vi "hmi-programming.vi"() -> ()   [LabVIEW 2017]
doc: "Demonstrates how to write and receive CAN frames via the Network Interface on the same port. \n\nTo write and receive frames via the Network Interface:\n- select the CAN Network Interface (i.e. CAN0, CAN1, etc.)\n- select the Baud Rate\n- run the VI\n- press the write button to write frames to the can bus\n\nEnable RTR Button to send a Remote Transmission Request or to simply send an empty Frame to request an Answer Frame from a connected device.\n\nEnable Extended Button to write extended Identifier Format. This is done by setting the 30th bit to enable extended format with the driver."
uses:
  <vilib>/nican/nican.llb/ncNetAttr.ctl
panel:
  in  "Tab Control":enum32{"Program", "Settings"}(tab)
  out "ID":u16 format="%04x"
  in  "Device":enum16{"Device 1", "Device 2"}(ring)
  out "Heartbeat":u16 format="%04x"
  in  "binFile":path
  in  "shutdown":bool
  in  "Initialize DFU":bool
  in  "Program":bool
  out "DFU Ready":bool
  out "Valid Path":bool
  out "Normal":bool
  in  "interface":string(combo)="CAN0" caption="Interface"
  # "PRESS AND HOLD"
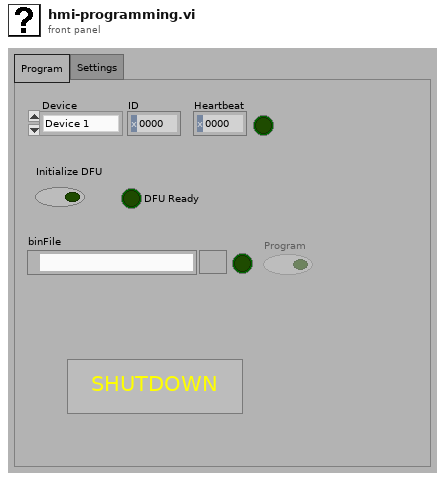
[diagram p1: front panel]
types:
  T1 = cluster{"Heartbeat":u16, "DFU":bool, "ValidPath":bool, "Path":path, "Normal":bool}
  T2 = typedef "ncNetAttr.ctl" = cluster{"Start On Open":enum32{"FALSE", "TRUE"}, "Baud Rate":u32, "Read Queue Length":u32, "Write Queue Length":u32, "Standard Comparator":u32, "Standard Mask":u32, "Extended Comparator":u32, "Extended Mask":u32}
  T3 = typedef "xobjhandle.ctl" = u32
  T4 = enum8{"Enabled", "Disabled", "Disabled and Grayed Out"}
  T5 = typedef "CanFrameTimed.ctl" = cluster{"Timestamp":dbl, "ArbitrationId":u32, "IsRemote":u8, "DataLength":u8, "Data":u8[]}
  T6 = cluster{dbl, u32, "IsRemote":u8, "DataLength":u8, u8[]}
  T7 = cluster{dbl, u32, "IsRemote":u8, "DataLength":u8, u8[]}[]
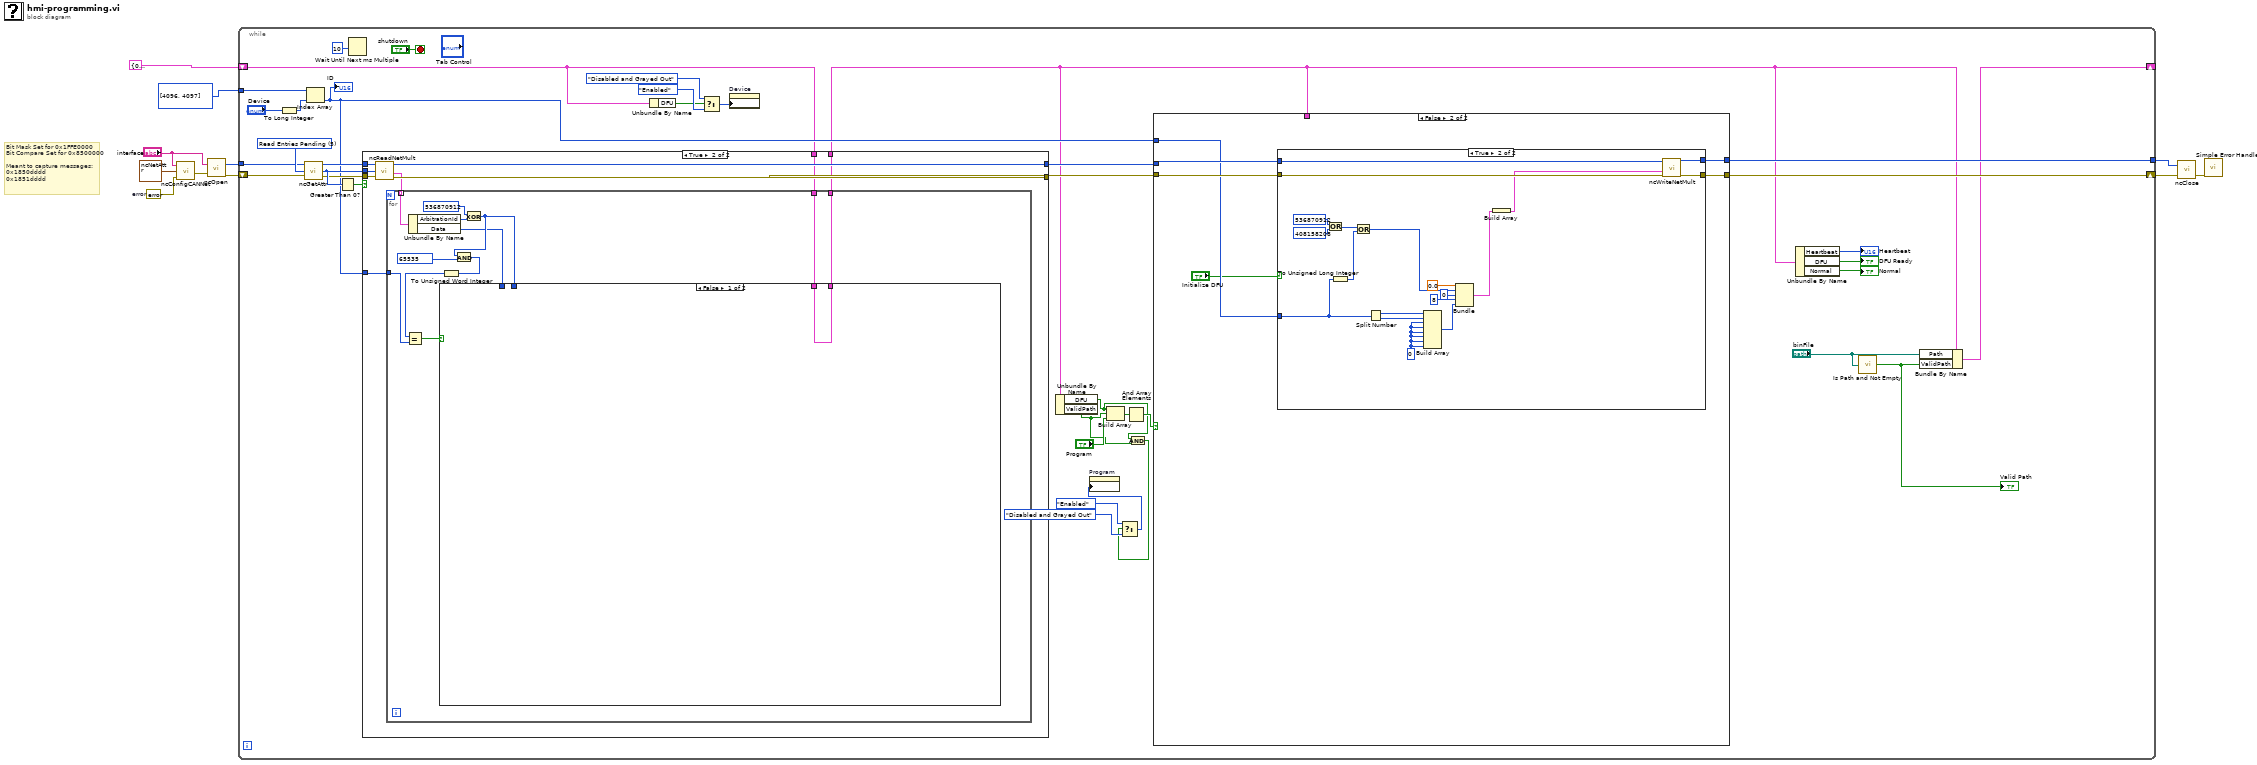
[diagram p0: block diagram]
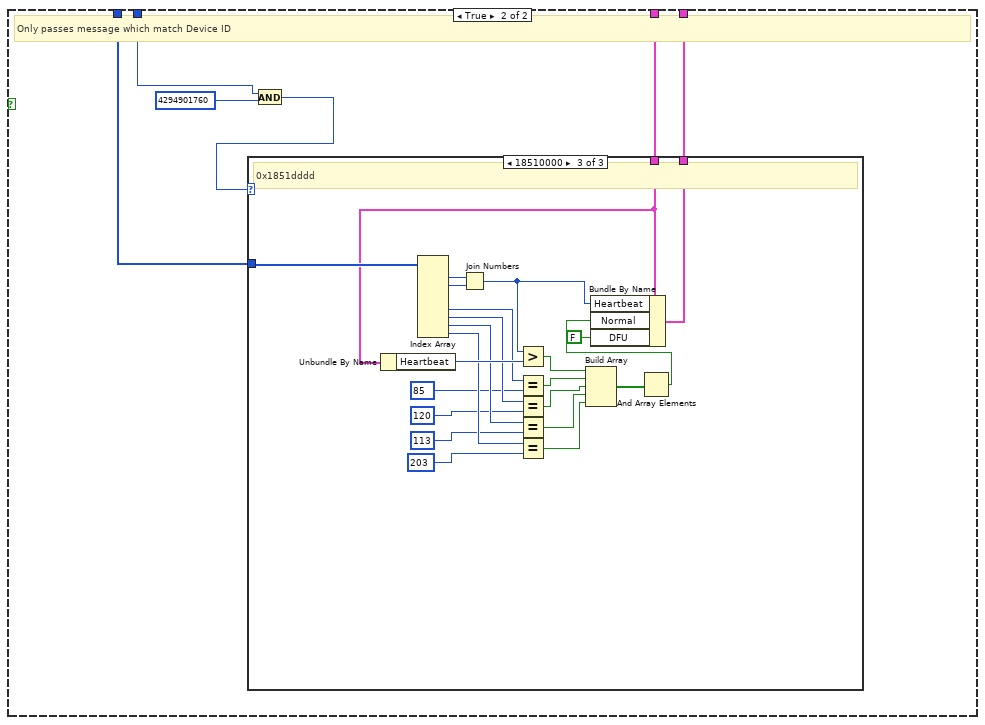
[diagram p3: hidden frame]
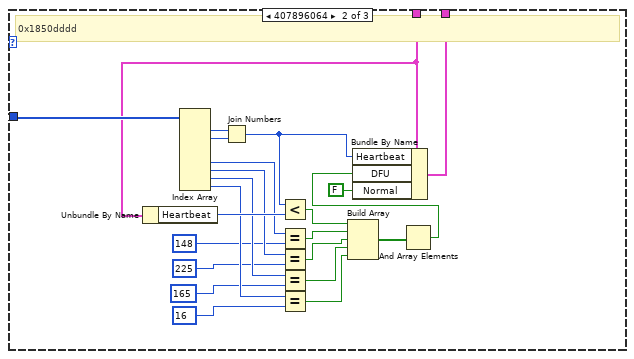
[diagram p5: hidden frame]
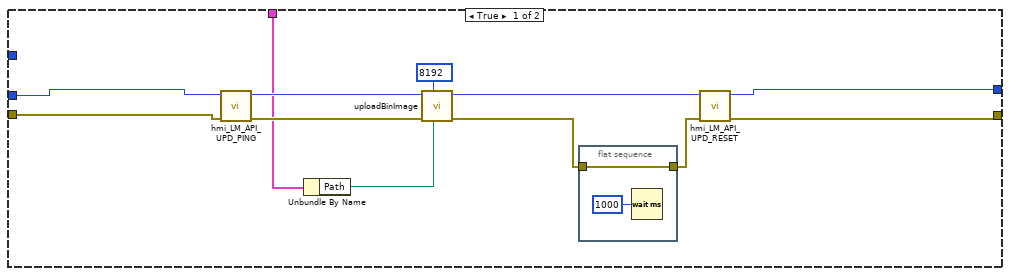
[diagram p6: hidden frame]
diagram:
  w7 = errorcluster {"status"=FALSE, "code"=0, "source"=""}  # error
  # "Bit Mask Set for 0x1FFE0000\nBit Compare Set for 0x8500000\n\nMeant to capture messages:\n0x1850dddd\n0x1851dddd"
  n1 = call <vilib>:"ncConfigCANNet.vi"("Error in"=w7, "CAN Network Interface Config"=T2 {"Start On Open"=enum."TRUE", "Baud Rate"=1000000, "Read Queue Length"=150, "Write Queue Length"=150, "Standard Comparator"=0, "Standard Mask"=0, "Extended Comparator"=407896064, "Extended Mask"=536739840}, "ObjName"="interface") -> ("Error out"=w8:errorcluster)  [unwired: 2 in]
  n2 = call <vilib>:"ncOpen.vi"("Error in"=w8, "ObjName"="interface") -> ("Error out"=w11:errorcluster, "ObjHandle out"=w9:T3)
  n3 = while {
    tunnel: w9 -> [w38]
    tunnel: [w48] -> w4
    shift-right: [w49] -> w3
    shift-left: w11 -> [w37]
    tunnel: u16[] [4096, 4097] -> [w36]
    shift-right: [w26] -> _
    shift-left: T1 {"Heartbeat"=0, "DFU"=FALSE, "ValidPath"=FALSE, "Path"=path "", "Normal"=FALSE} -> [w19]
    stop <- "shutdown" stop-if-true
    w41 = u32 5 items=["(reserved)", "Protocol Version", "Software Version", "Object State", "(reserved)", "Read Entries Pending", "Write Entries Pending", "ReadMult Size for Notification", "Listen Only?", "Self Reception?", "Transmit Error Counter", "Receive Error Counter", "Single Shot Transmit?", "Series 2 Filter Mode", "Series 2 Mask", "Series 2 Comparator", "Serial Number", "Form Factor", "Series", "Transceiver Type", "Interface Number", "Series 2 Error/Arb Capture", "Transceiver Mode", "Transceiver External Outputs", "Transceiver External Inputs", "Start Trigger Behavior", "Log Comm Warnings", "User RTSI Frame", "Transmit Mode", "Log Start Trigger?", "Timestamp Format", "Master Timebase Rate", "Virtual Bus Timing"] ("AttrId")
    n4 = To Long Integer(number="Device") -> (32bit integer=w34:i32)
    n5 = call <vilib>:"ncGetAttr.vi"("Error in"=w37, "AttrId"=w41, "ObjHandle in"=w38) -> ("Error out"=w42:errorcluster, "AttrValue"=w45:u32, "ObjHandle out"=w43:T3)
    n6 = Index Array(array=w36, index=w34) -> (element=w33:u16)
    "ID" <- w33
    n7 = Greater Than 0?(x=w45) -> (x > 0?=w44:bool)
    n8 = Wait Until Next ms Multiple(millisecond multiple=u32 10) -> ()  [unwired: 1 out]
    n9 = case shown="True" w44 {
      tunnel: [w51 w61] -> w39
      tunnel: [w52 w60] -> w40
      tunnel: w45 -> [_ w59]
      tunnel: w42 -> [w51 w58]
      tunnel: w43 -> [w52 w57]
      tunnel: w33 -> [_ w55]
      tunnel: w19 -> [w50 w54]
      tunnel: [w50 w53] -> w27
      frame False {
      }
      frame True {
        n10 = call <vilib>:"ncReadNetMult.vi"("ObjHandle in"=w57, "Requested Number of Frames"=w59, "Error in"=w58) -> ("ObjHandle out"=w60:T3, "Data"=w56:T5[], "Error out"=w61:errorcluster)  [unwired: 1 out]
        n11 = for {
          tunnel: w56 -> [w73] mode=indexing
          tunnel: w55 -> [w70]
          tunnel: w54 -> [w64]
          tunnel: [w63] -> w53
          n12 = Unbundle By Name(w73) -> ("ArbitrationId"=w71:u32, "Data"=w66:u8[])
          n13 = Exclusive Or(1:w71, 2:u32 536870912 ("y")) -> (0:w67:u32)
          n14 = And(x=w67, y=u32 65535) -> (x .and. y?=w69:u32)
          n15 = To Unsigned Word Integer(number=w69) -> (unsigned 16bit integer=w65:u16)
          n16 = Equal?(x=w65, y=w70) -> (x = y?=w68:bool)
          n17 = case shown="False" w68 {
            tunnel: w67 -> [_ w75]
            tunnel: w66 -> [_ w80]
            tunnel: w64 -> [w74 w78]
            tunnel: [w74 w77] -> w63
            frame False {
            }
            frame True {
              # "Only passes message which match Device ID"
              n18 = And(x=w75, y=u32 4294901760) -> (x .and. y?=w79:u32)
              n19 = case shown="18510000" w79 {
                tunnel: w80 -> [_ w102 w125]
                tunnel: w78 -> [w81 w100 w123]
                tunnel: [w81 w101 w124] -> w77
                frame Default {
                }
                frame 407896064 {
                  # "0x1850dddd"
                  n20 = Unbundle By Name(w100) -> ("Heartbeat"=w99:u16)
                  n21 = Index Array(array=w102) -> (element #1=w103:u8, element #2=w104:u8, element #5=w92:u8, element #6=w91:u8, element #7=w90:u8, element #8=w89:u8)  [unwired: 8 in, 2 out]
                  n22 = Join Numbers(hi=w103, lo=w104) -> ((hi.lo)=w98:u16)
                  n23 = Less?(x=w98, y=w99) -> (x < y?=w97:bool)
                  n24 = Equal?(x=w92, y=u8 148) -> (x = y?=w96:bool)
                  n25 = Equal?(x=w91, y=u8 225) -> (x = y?=w95:bool)
                  n26 = Equal?(x=w90, y=u8 165) -> (x = y?=w94:bool)
                  n27 = Equal?(x=w89, y=u8 16) -> (x = y?=w93:bool)
                  n28 = Build Array(w97, w96, w95, w94, w93) -> (w84:bool[])
                  n29 = And Array Elements(Boolean array=w84) -> (logical AND=w83:bool)
                  n30 = Bundle By Name(cluster=w100, "Heartbeat"=w98, "DFU"=w83, "Normal"=FALSE) -> (w101:T1)
                }
                frame 407961600 {
                  # "0x1851dddd"
                  n31 = Unbundle By Name(w123) -> ("Heartbeat"=w122:u16)
                  n32 = Index Array(array=w125) -> (element #1=w126:u8, element #2=w127:u8, element #5=w115:u8, element #6=w114:u8, element #7=w113:u8, element #8=w112:u8)  [unwired: 8 in, 2 out]
                  n33 = Join Numbers(hi=w126, lo=w127) -> ((hi.lo)=w121:u16)
                  n34 = Greater?(x=w121, y=w122) -> (0:w120:bool)
                  n35 = Equal?(x=w115, y=u8 85) -> (x = y?=w119:bool)
                  n36 = Equal?(x=w114, y=u8 120) -> (x = y?=w118:bool)
                  n37 = Equal?(x=w113, y=u8 113) -> (x = y?=w117:bool)
                  n38 = Equal?(x=w112, y=u8 203) -> (x = y?=w116:bool)
                  n39 = Build Array(w120, w119, w118, w117, w116) -> (w107:bool[])
                  n40 = And Array Elements(Boolean array=w107) -> (logical AND=w106:bool)
                  n41 = Bundle By Name(cluster=w123, "Heartbeat"=w121, "Normal"=w106, "DFU"=FALSE) -> (w124:T1)
                }
              }
            }
          }
        }
      }
    }
    n42 = Unbundle By Name(w19) -> ("DFU"=w18:bool)
    n43 = Select(t=T4."Disabled and Grayed Out" ("Disabled"), s=w18, f=T4."Enabled" ("Disabled")) -> (s? t:f=w20:T4)
    n44 = property on="Device" class="Enum (strict)"("DisabledEnum"=w20) -> ()  [unwired: 2 in, 2 out]
    n45 = Unbundle By Name(w27) -> ("DFU"=w14:bool, "ValidPath"=w13:bool)
    n46 = Build Array(w14, w13, "Program") -> (w29:bool[])
    n47 = And Array Elements(Boolean array=w29) -> (logical AND=w28:bool)
    n48 = And(x=w14, y=w13) -> (x .and. y?=w12:bool)
    n49 = Select(t=T4."Enabled" ("Disabled"), s=w12, f=T4."Disabled and Grayed Out" ("Disabled")) -> (s? t:f=w15:T4)
    n50 = property on="Program" class="Bool"("DisabledEnum"=w15) -> ()  [unwired: 2 in, 2 out]
    n51 = case shown="False" w28 {
      tunnel: [w130 w147] -> w49
      tunnel: [w131 w146] -> w48
      tunnel: w40 -> [w133 w145]
      tunnel: w39 -> [w132 w144]
      tunnel: w33 -> [_ w143]
      tunnel: w27 -> [w129 _]
      frame True {
        n52 = call "hmi_LM_API_UPD_PING.vi"("Error in"=w132, "canSession"=w133) -> ("Error out"=w137:errorcluster, "canSession"=w138:T3)  [unwired: 7 in, 1 out]
        n53 = Unbundle By Name(w129) -> ("Path"=w128:path)
        n54 = call "uploadBinImage.vi"("binFile"=w128, "dloadAddr"=u32 8192 ("dloadSize"), "Error in"=w137, "canSession"=w138) -> ("Error out"=w136:errorcluster, "canSession"=w135:T3)  [unwired: 5 in, 1 out]
        n55 = flat-sequence {
          tunnel: w136 -> [w141]
          tunnel: [w141] -> w139
          frame #0 {
            n56 = Wait (ms)(milliseconds to wait=u32 1000) -> ()  [unwired: 1 out]
          }
        }
        n57 = call "hmi_LM_API_UPD_RESET.vi"("Error in"=w139, "canSession"=w135) -> ("Error out"=w130:errorcluster, "canSession"=w131:T3)  [unwired: 8 in]
      }
      frame False {
        n58 = case shown="True" "Initialize DFU" {
          tunnel: [w148 w168] -> w147
          tunnel: [w149 w167] -> w146
          tunnel: w145 -> [w149 w166]
          tunnel: w144 -> [w148 w165]
          tunnel: w143 -> [_ w153]
          frame False {
          }
          frame True {
            w164 = u8 0
            n59 = Or(x=u32 536870912 ("y"), y=u32 408158208) -> (x .or. y?=w151:u32)
            n60 = To Unsigned Long Integer(number=w153) -> (unsigned 32bit integer=w152:u32)
            n61 = Or(x=w151, y=w152) -> (x .or. y?=w150:u32)
            n62 = Split Number(x=w153) -> (hi(x)=w157:u8, lo(x)=w156:u8)
            n63 = Build Array(w157, w156, w164, w164, w164, w164, w164, w164) -> (w162:u8[])
            n64 = Bundle(0.0, w150, "IsRemote"=u8 0, "DataLength"=u8 8, w162) -> (w155:T6)  [unwired: 1 in]
            n65 = Build Array(w155) -> (w154:T7)
            n66 = call <vilib>:"ncWriteNetMult.vi"("Error in"=w165, "Data"=w154, "ObjHandle in"=w166) -> ("Error out"=w168:errorcluster, "ObjHandle out"=w167:T3)  [unwired: 7 in]
          }
        }
      }
    }
    n67 = Unbundle By Name(w27) -> ("Heartbeat"=→"Heartbeat":u16, "DFU"=→"DFU Ready":bool, "Normal"=→"Normal":bool)
    n68 = call <vilib>:"Is Path and Not Empty.vi"("path"="binFile") -> ("Is Path and Not Empty?"=w24:bool)  [unwired: 4 in]
    "Valid Path" <- w24
    n69 = Bundle By Name(cluster=w27, "Path"="binFile", "ValidPath"=w24) -> (w26:T1)
  }
  n70 = call <vilib>:"ncClose.vi"("Error in"=w3, "ObjHandle in"=w4) -> ("Error out"=w5:errorcluster)  [unwired: 1 in]
  n71 = call <vilib>:"Simple Error Handler.vi"("error in (no error)"=w5) -> ()  [unwired: 4 in, 5 out]
